vi "testCamera.vi"() -> ()   [LabVIEW 2015]
uses:
  <vilib>/userdefined/High Color/IMAQdx.ctl
  <vilib>/Utility/file.llb/Write To Spreadsheet File (DBL).vi
  <vilib>/Utility/file.llb/Write To Spreadsheet File (string).vi
  <vilib>/vision/driver/NI_Vision_Acquisition_Software.lvlib
  <resource>/objmgr/imaqdx.rc
panel:
  out "appended array":dbl[](array[numeric])
  in  "step y":dbl
  in  "step x":dbl
  in  "y":dbl
  in  "x":dbl
  in  "add":bool
  in  "Channel Names":string[](array[string])=["Channel 1", "Channel 2", "Channel 3", "Channel 4", "Channel 5"]
  in  "File Name":path=path "C:/Documents and Settings/husmith/Desktop/CSVdata.csv"
  out "Circles":cluster{"x":dbl, "y":dbl, "r":dbl}[](array[cluster])
  out "Image 2":T1(plugin-control)
  out "Circles (Shape Detection 1)":T2(array[cluster]) {"Position"."Y" format="%.2f"; "Position"."X" format="%.2f"}
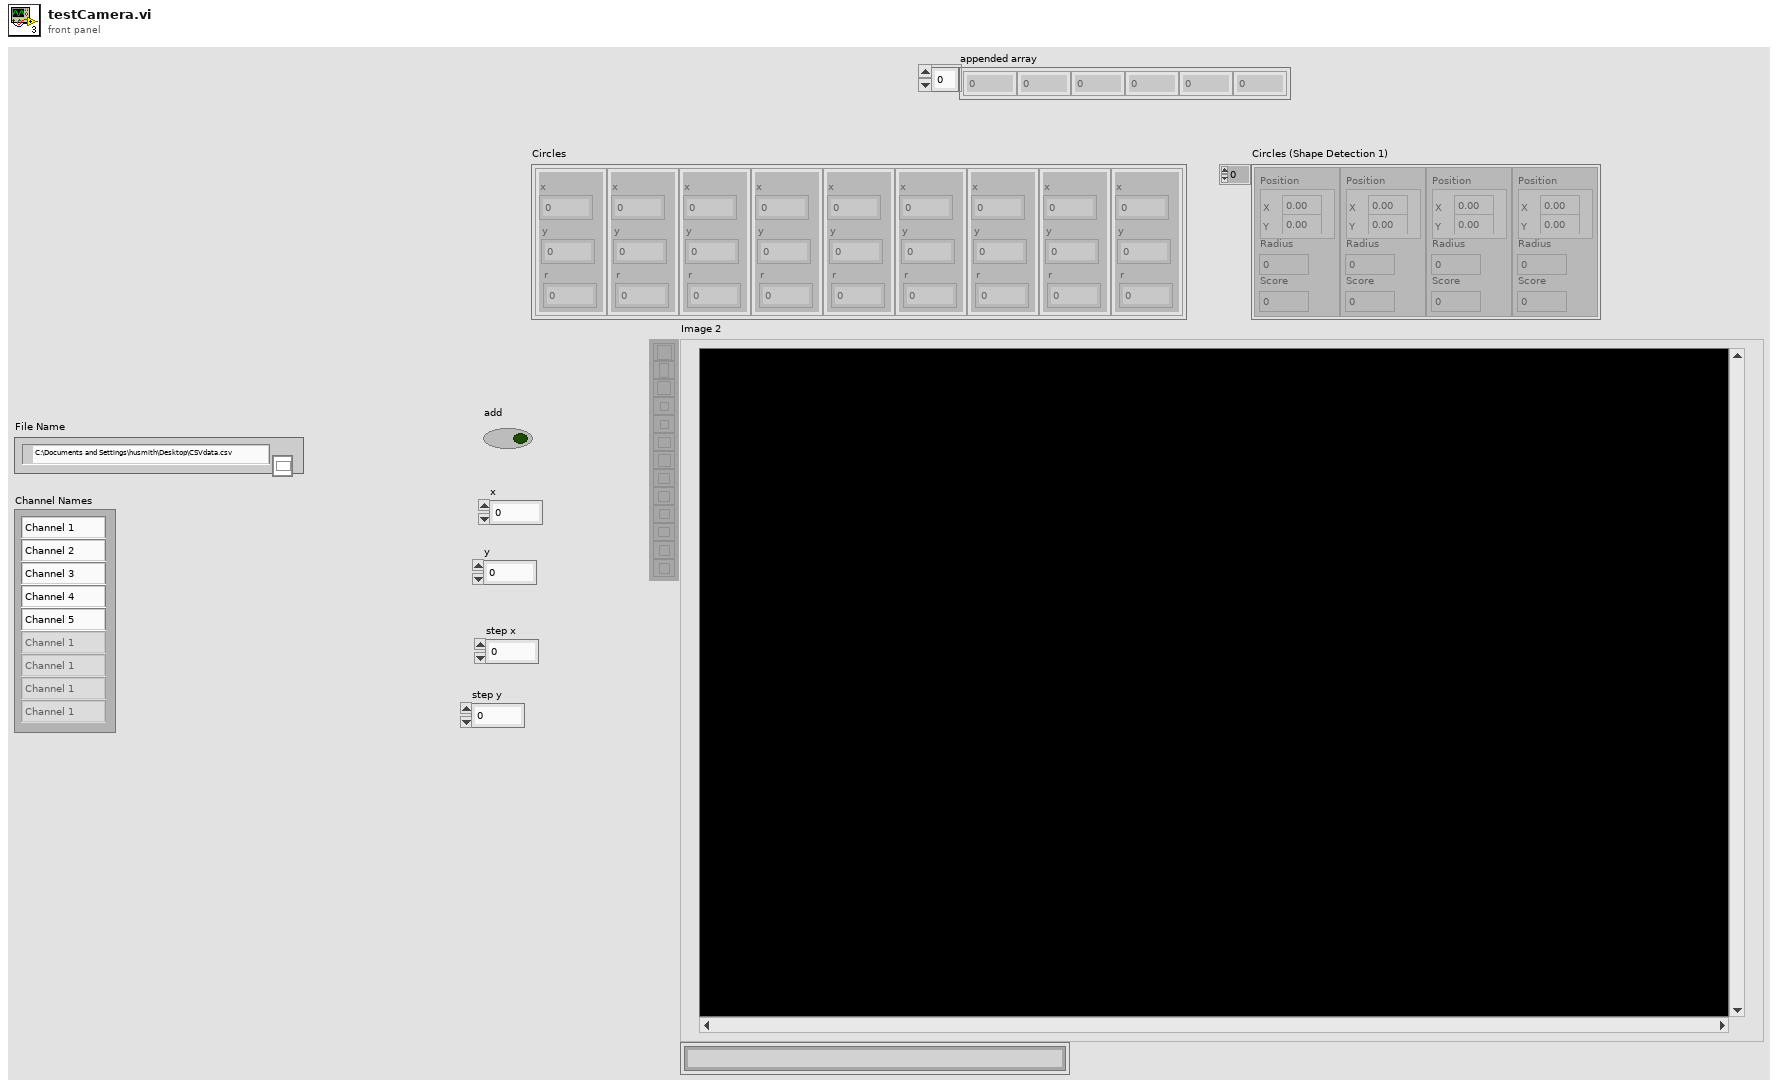
[diagram p1: front panel]
types:
  T1 = typedef "IMAQ Image.ctl" = refnum<image>
  T2 = cluster{"Position":cluster{"X":sgl, "Y":sgl}, "Radius":dbl, "Score":dbl}[]
  T3 = typedef "IMAQdx.ctl" = refnum<k21>
  T4 = cluster{"Position":cluster{"X":sgl, "Y":sgl}, "Radius":dbl, "Score":dbl}
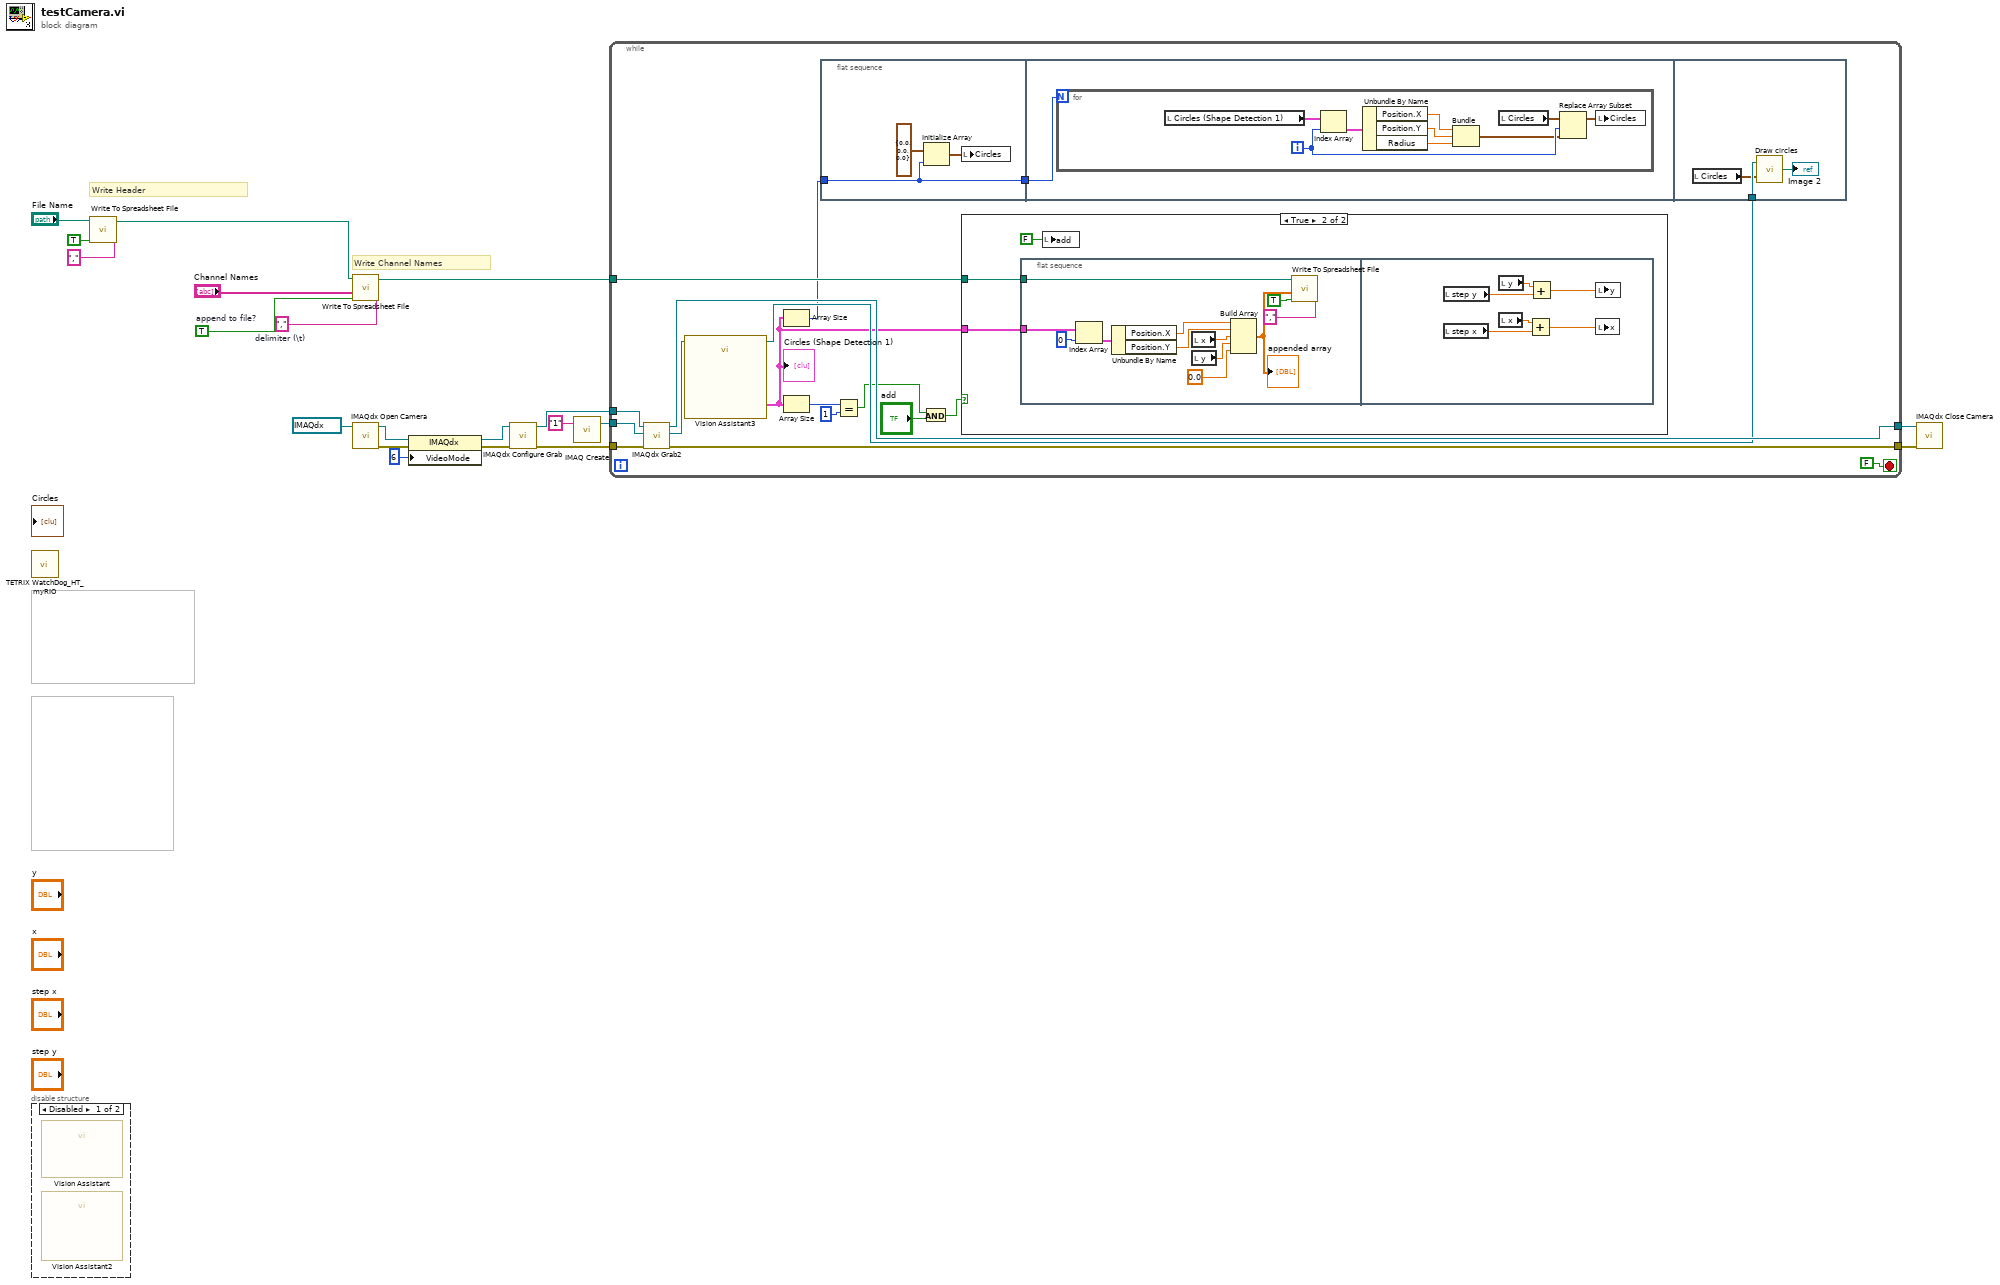
[diagram p0: block diagram]
diagram:
  w5 = TRUE  # append to file?
  w4 = ","  # delimiter (\t)
  # "Write Header"
  # "Write Channel Names"
  n1 = call <vilib>:"TETRIX WatchDog_HT_myRIO.vi"() -> ()  [unwired: 3 in, 1 out]
  n2 = disable-structure shown="Disabled" {
    frame Disabled {
      n3 = call "Vision Assistant"() -> ()  [unwired: 26 in, 2 out]
      n4 = call "Vision Assistant2"() -> ()  [unwired: 26 in, 2 out]
    }
    frame Enabled {
    }
  }
  n5 = call-poly <vilib>:"Write To Spreadsheet File.vi"("delimiter (\\t)"="," ("delimiter (\\t)"), "append to file? (new file:F)"=TRUE, "file path (dialog if empty)"="File Name") -> ("new file path (Not A Path if cancelled)"=w3:path)  [unwired: 4 in, 1 out]
  n6 = call-poly <vilib>:"Write To Spreadsheet File.vi"("delimiter (\\t)"=w4, "append to file? (new file:F)"=w5, "1D data"="Channel Names", "file path (dialog if empty)"=w3) -> ("new file path (Not A Path if cancelled)"=w1:path)  [unwired: 3 in, 1 out]
  n7 = call <vilib>:"IMAQdx Open Camera.vi"("Session In"=T3 "cam0") -> ("error out"=w12:errorcluster, "Session Out"=w13:T3)  [unwired: 9 in]
  n8 = property class="IMAQdx"(reference=w13, error in=w12, "VideoMode"=u32 6) -> (reference out=w10:T3, error out=w11:errorcluster)
  n9 = call <vilib>:"IMAQdx Configure Grab.vi"("error in"=w11, "Session In"=w10) -> ("error out"=w19:errorcluster, "Session Out"=w18:T3)  [unwired: 8 in]
  n10 = call "IMAQ Create"("Image Name"="1") -> ("New Image"=w16:T1)  [unwired: 4 in, 1 out]
  n11 = while {
    tunnel: w19 -> [w37]
    tunnel: w18 -> [w36]
    tunnel: [w35] -> w17
    tunnel: w16 -> [w34]
    tunnel: [w33] -> w14
    tunnel: w1 -> [w28]
    stop <- FALSE stop-if-true
    n12 = call <vilib>:"IMAQdx Grab2.vi"("error in"=w37, "Image In"=w34, "Session In"=w36) -> ("error out"=w33:errorcluster, "Image Out"=w31:T1, "Session Out"=w35:T3)  [unwired: 5 in, 1 out]
    n13 = call "Vision Assistant3"("Image In"=w31) -> ("Image Out"=w30:T1, "Circles (Shape Detection 1)"=w21:T2)  [unwired: 24 in, 1 out]
    "Circles (Shape Detection 1)" <- w21
    n14 = Array Size(array=w21) -> (size(s)=w22:i32)
    n15 = Array Size(array=w21) -> (size(s)=w27:i32)
    n16 = flat-sequence {
      tunnel: [w61] -> w29
      tunnel: w22 -> [w61]
      tunnel: w29 -> [w62]
      tunnel: w30 -> [w73]
      frame #0 {
        n17 = Initialize Array(cluster{"x":dbl, "y":dbl, "r":dbl} {"x"=0.0, "y"=0.0, "r"=0.0} ("circle"), w61) -> (w60:cluster{"x":dbl, "y":dbl, "r":dbl}[])
        n18 = local write "Circles"(w60) -> ()
      }
      frame #1 {
        n19 = for {
          N: w62 -> [_]
          i -> [w65]
          n20 = local read "Circles (Shape Detection 1)"() -> (w71:T2)
          n21 = Index Array(array=w71, index=w65) -> (element=w70:T4)
          n22 = Unbundle By Name(w70) -> ("Position.X"=w69:sgl, "Position.Y"=w68:sgl, "Radius"=w67:dbl)
          n23 = Bundle("X"=w69, "Y"=w68, "Radius"=w67) -> (w64:cluster{"X":sgl, "Y":sgl, "Radius":dbl})  [unwired: 1 in]
          n24 = local read "Circles"() -> (w66:cluster{"x":dbl, "y":dbl, "r":dbl}[])
          n25 = Replace Array Subset(array=w66, new element=w64, index=w65) -> (w63:cluster{"x":dbl, "y":dbl, "r":dbl}[])
          n26 = local write "Circles"(w63) -> ()
        }
      }
      frame #2 {
        n27 = local read "Circles"() -> (w72:cluster{"x":dbl, "y":dbl, "r":dbl}[])
        n28 = call "Draw circles .vi"("Circles"=w72, "Refnum in"=w73) -> ("Refnum out"=→"Image 2":T1)
      }
    }
    n29 = Equal?(x=w27, y=1) -> (x = y?=w25:bool)
    n30 = And(x=w25, y="add") -> (x .and. y?=w23:bool)
    n31 = case shown="True" w23 {
      tunnel: w21 -> [_ w40]
      tunnel: w28 -> [_ w39]
      frame False {
      }
      frame True {
        n32 = flat-sequence {
          tunnel: w40 -> [w45]
          tunnel: w39 -> [w44]
          frame #0 {
            n33 = Index Array(array=w45, index=0) -> (element=w50:T4)
            n34 = Unbundle By Name(w50) -> ("Position.X"=w48:sgl, "Position.Y"=w47:sgl)
            n35 = local read "x"() -> (w43:dbl)
            n36 = local read "y"() -> (w42:dbl)
            n37 = Build Array(w48, w47, w43, w42, 0.0 ("element")) -> (w46:dbl[])
            "appended array" <- w46
            n38 = call-poly <vilib>:"Write To Spreadsheet File.vi"("delimiter (\\t)"="," ("delimiter (\\t)"), "append to file? (new file:F)"=TRUE, "1D data"=w46, "file path (dialog if empty)"=w44) -> ()  [unwired: 3 in, 2 out]
          }
          frame #1 {
            n39 = local read "step y"() -> (w54:dbl)
            n40 = local read "step x"() -> (w57:dbl)
            n41 = local read "y"() -> (w55:dbl)
            n42 = local read "x"() -> (w58:dbl)
            n43 = Add(x=w58, y=w57) -> (x+y=w56:dbl)
            n44 = Add(x=w55, y=w54) -> (x+y=w53:dbl)
            n45 = local write "y"(w53) -> ()
            n46 = local write "x"(w56) -> ()
          }
        }
        n47 = local write "add"(FALSE ("add")) -> ()
      }
    }
  }
  n48 = call <vilib>:"IMAQdx Close Camera.vi"("error in"=w14, "Session In"=w17) -> ()  [unwired: 9 in, 1 out]
